vi "Scale_DiodeTemp.vi"(4 "uTTA_MetaData_in":T2 {"No Suspect Lines" format="%.3pV"; "Interpolation Factor m" format="%.2g"; "Interpolation Offset" format="%.2g"; "Chip Size" format="%.2gmm²"; "Heating Power" format="%.3pW"; "Cool Volt Deviation" format="%.3pV"; "Cool Voltage" format="%.3pV"; "Tsamp,fast" format="%#_3gus"; "Tsamp,slow" format="%#_3gus"; "T_Preheat" format="%#_3gs"; "T_Heat" format="%#_3gs"; "T_Cool" format="%#_3gs"}, 5 "uTTA_MeasData_in":T1, 7 "DUT Settings":T3) -> (1 "uTTA_MeasData_out":T1, 2 "Diode Cold Temp":dbl)   [LabVIEW 2021]
uses:
  CTRL_DUT_SETTINGS.ctl
  uTTA_MetaData.ctl
  CTL_uTTA_MeasurementData.ctl
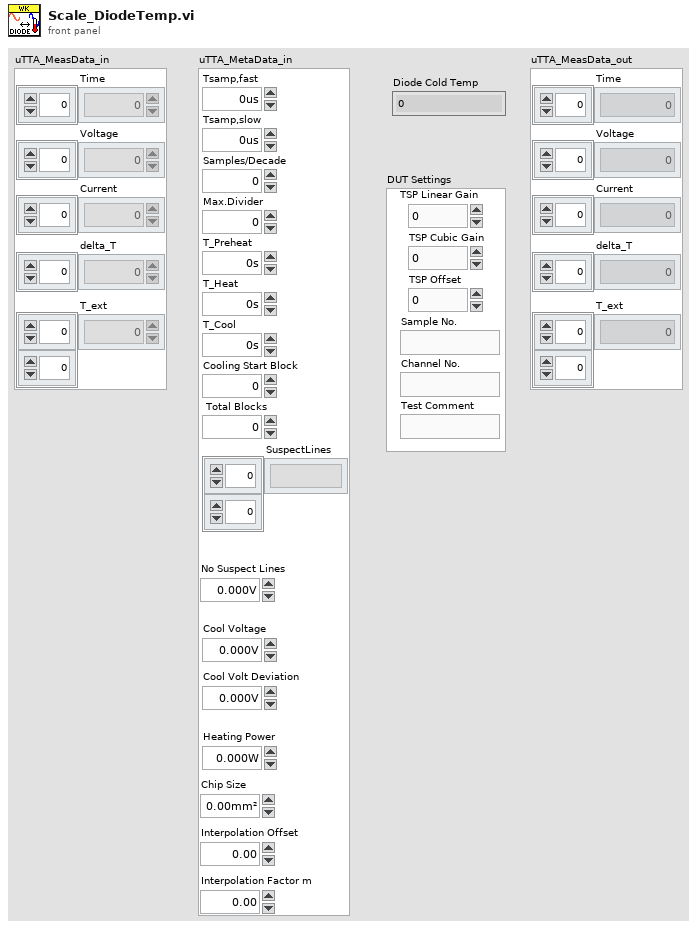
[diagram p1: front panel]
types:
  T1 = typedef "CTL_uTTA_MeasurementData.ctl" = cluster{"Time":dbl[], "Voltage":dbl[], "Current":dbl[], "delta_T":dbl[], "T_ext":dbl[][]}
  T2 = typedef "uTTA_MetaData.ctl" = cluster{"Tsamp,fast":dbl, "Tsamp,slow":dbl, "Samples/Decade":u32, "Max.Divider":u32, "T_Preheat":dbl, "T_Heat":dbl, "T_Cool":dbl, "Cooling Start Block":u32, " Total Blocks":u32, "SuspectLines":string[][], "Cool Voltage":dbl, "Cool Volt Deviation":dbl, "Heating Power":dbl, "Chip Size":dbl, "Interpolation Offset":dbl, "Interpolation Factor m":dbl, "No Suspect Lines":u32}
  T3 = typedef "CTRL_DUT_SETTINGS.ctl" = cluster{"Test Comment":string, "Channel No.":string, "Sample No.":string, "TSP Offset":dbl, "TSP Cubic Gain":dbl, "TSP Linear Gain":dbl}
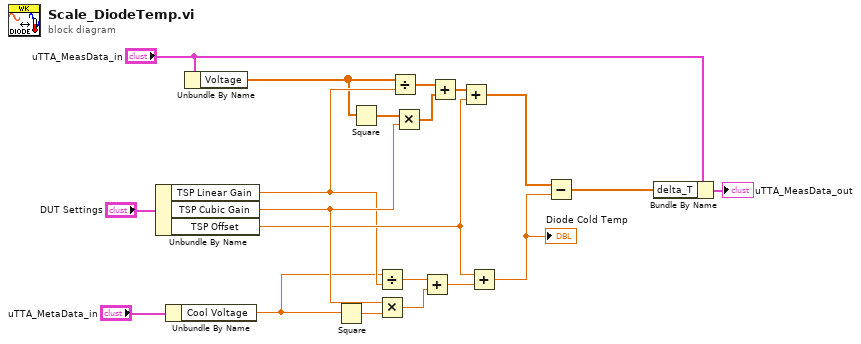
[diagram p0: block diagram]
diagram:
  n1 = Unbundle By Name("DUT Settings") -> ("TSP Linear Gain"=w7:dbl, "TSP Cubic Gain"=w12:dbl, "TSP Offset"=w11:dbl)
  n2 = Unbundle By Name("uTTA_MetaData_in") -> ("Cool Voltage"=w2:dbl)
  n3 = Unbundle By Name("uTTA_MeasData_in") -> ("Voltage"=w6:dbl[])
  n4 = Square(x=w2) -> (x^2=w14:dbl)
  n5 = Square(x=w6) -> (x^2=w19:dbl[])
  n6 = Divide(x=w2, y=w7) -> (x/y=w13:dbl)
  n7 = Multiply(x=w12, y=w14) -> (x*y=w15:dbl)
  n8 = Divide(x=w6, y=w7) -> (x/y=w20:dbl[])
  n9 = Multiply(x=w19, y=w12) -> (x*y=w18:dbl[])
  n10 = Add(x=w13, y=w15) -> (x+y=w16:dbl)
  n11 = Add(x=w20, y=w18) -> (x+y=w17:dbl[])
  n12 = Add(x=w17, y=w11) -> (x+y=w9:dbl[])
  n13 = Add(x=w11, y=w16) -> (x+y=w10:dbl)
  "Diode Cold Temp" <- w10
  n14 = Subtract(x=w9, y=w10) -> (x-y=w4:dbl[])
  n15 = Bundle By Name(cluster="uTTA_MeasData_in", "delta_T"=w4) -> (→"uTTA_MeasData_out":T1)
